vi "ValueAsString.vi"(8 "error in (no error)":errorcluster, 11 "Parameter":string="  <value><string>RHAT</string></value>\n    ") -> (0 "error out":errorcluster, 3 "value":string)   [LabVIEW 2009]
doc: "Convert XML-RPC formatted string to LV string"
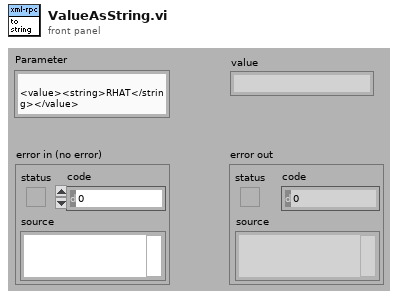
[diagram p1: front panel]
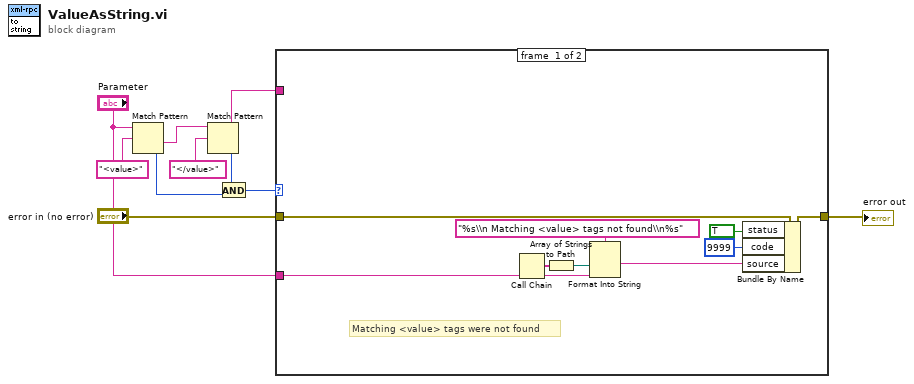
[diagram p0: block diagram]
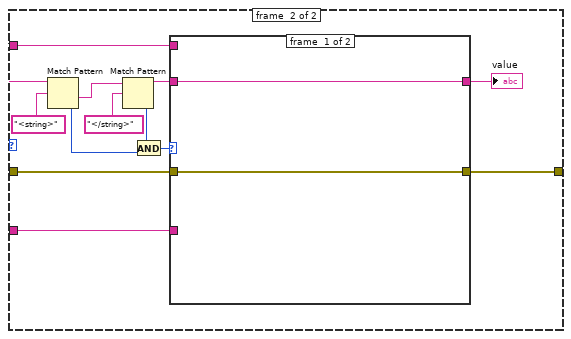
[diagram p2: hidden frame]
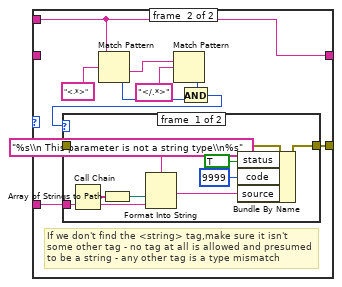
[diagram p3: hidden frame]
diagram:
  n1 = Match Pattern(string="Parameter", regular expression="<value>") -> (after substring=w9:string, offset past match=w2:i32)  [unwired: 1 in, 2 out]
  n2 = Match Pattern(string=w9, regular expression="</value>") -> (before substring=w7:string, offset past match=w3:i32)  [unwired: 1 in, 2 out]
  n3 = And(x=w3, y=w2) -> (x .and. y?=w1:i32)
  n4 = case shown="Default" w1 {
    tunnel: w7 -> [_ w28]
    tunnel: "error in (no error)" -> [w13 w26]
    tunnel: [w12 w24] -> w5
    tunnel: "Parameter" -> [w16 w23]
    frame #0 {
      # "Matching <value> tags were not found"
      n5 = Call Chain() -> (call chain=w19:string[])
      n6 = Array of Strings to Path(0:w19) -> (2:w18:path)  [unwired: 1 in]
      n7 = Format Into String(format string="%s\\n Matching <value> tags not found\\n%s", w18, w16) -> (resulting string=w11:string)  [unwired: 2 in, 1 out]
      n8 = Bundle By Name(cluster=w13, "status"=TRUE, "code"=9999, "source"=w11) -> (w12:errorcluster)
    }
    frame #1 {
      n9 = Match Pattern(string=w28, regular expression="<string>") -> (after substring=w30:string, offset past match=w21:i32)  [unwired: 1 in, 2 out]
      n10 = Match Pattern(string=w30, regular expression="</string>") -> (before substring=w27:string, offset past match=w22:i32)  [unwired: 1 in, 2 out]
      n11 = And(x=w22, y=w21) -> (x .and. y?=w20:i32)
      n12 = case shown="-1" w20 {
        tunnel: w28 -> [_ w34]
        tunnel: w27 -> [w33 _]
        tunnel: [w33 w34] -> w25
        tunnel: w26 -> [w32 w40]
        tunnel: [w32 w39] -> w24
        tunnel: w23 -> [_ w38]
        frame #0 {
        }
        frame #1 {
          # "If we don't find the <string> tag,make sure it isn't some other tag - no tag at all is allowed and presumed to be a string - any other tag is a type mismatch"
          n13 = Match Pattern(string=w34, regular expression="<.*>") -> (after substring=w42:string, offset past match=w35:i32)  [unwired: 1 in, 2 out]
          n14 = Match Pattern(string=w42, regular expression="</.*>") -> (offset past match=w36:i32)  [unwired: 1 in, 3 out]
          n15 = And(x=w36, y=w35) -> (x .and. y?=w37:i32)
          n16 = case shown="-1" w37 {
            tunnel: w40 -> [w51 w53]
            tunnel: [w50 w53] -> w39
            tunnel: w38 -> [w45 _]
            frame #0 {
              n17 = Call Chain() -> (call chain=w52:string[])
              n18 = Array of Strings to Path(0:w52) -> (2:w47:path)  [unwired: 1 in]
              n19 = Format Into String(format string="%s\\n This parameter is not a string type\\n%s", w47, w45) -> (resulting string=w46:string)  [unwired: 2 in, 1 out]
              n20 = Bundle By Name(cluster=w51, "status"=TRUE, "code"=9999, "source"=w46) -> (w50:errorcluster)
            }
            frame #1 {
            }
          }
        }
      }
      "value" <- w25
    }
  }
  "error out" <- w5
